vi "Parse GID_Telemetry.vi"(10 "Data In":variant) -> (2 "GID Telemetry":T1 {"Register_1"."A_Angle" format="%04x"; "Register_1"."B_Angle" format="%04x"; "Register_2"."Read_Time" format="%d ms"; "Register_2"."CMD_Code" format="%.0x"; "Register_2"."Head_Sel" format="%.0x"; "Register_7"."Spare" format="%04x"; "Register_8"."Spare" format="%04x"; "Register_A"."Spare" format="%04x"})   [LabVIEW 2019]
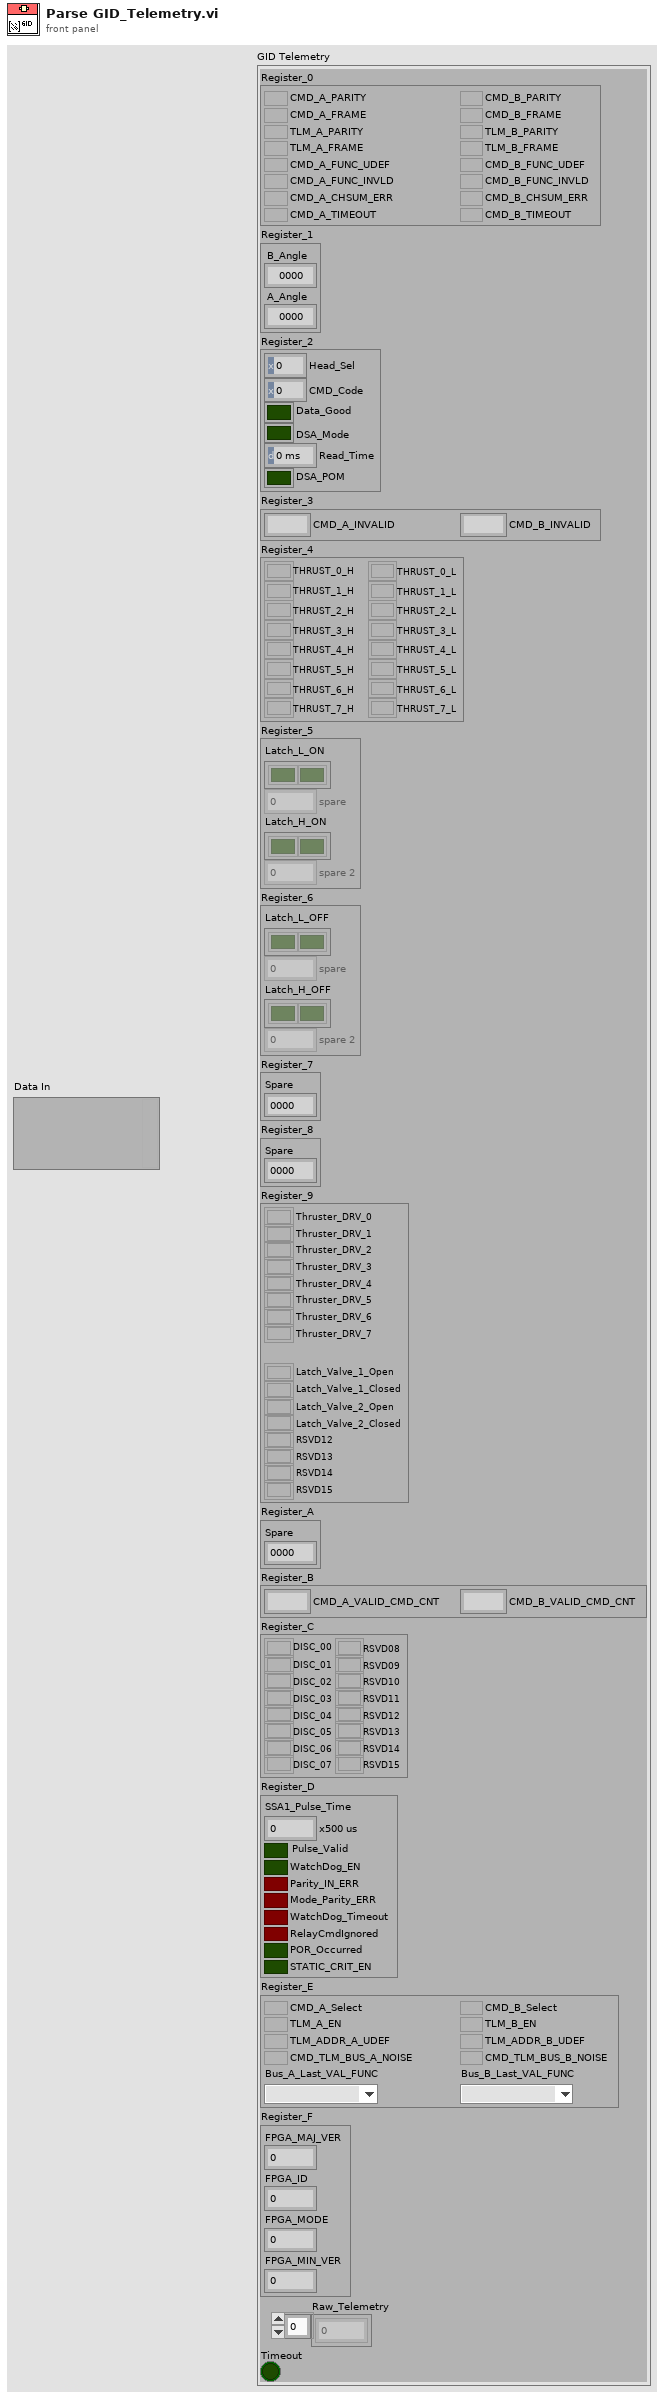
[diagram p1: front panel]
types:
  T1 = cluster{"Register_0":cluster{"CMD_B_PARITY":bool, "CMD_A_PARITY":bool, "CMD_B_FRAME":bool, "CMD_A_FRAME":bool, "TLM_B_PARITY":bool, "TLM_A_PARITY":bool, "TLM_B_FRAME":bool, "TLM_A_FRAME":bool, "CMD_B_FUNC_UDEF":bool, "CMD_A_FUNC_UDEF":bool, "CMD_B_FUNC_INVLD":bool, "CMD_A_FUNC_INVLD":bool, "CMD_B_CHSUM_ERR":bool, "CMD_A_CHSUM_ERR":bool, "CMD_B_TIMEOUT":bool, "CMD_A_TIMEOUT":bool}, "Register_1":cluster{"B_Angle":u8, "A_Angle":u8}, "Register_2":cluster{"Head_Sel":u8, "CMD_Code":u8, "Data_Good":bool, "DSA_Mode":bool, "Read_Time":u8, "DSA_POM":bool}, "Register_3":cluster{"CMD_B_INVALID":u8, "CMD_A_INVALID":u8}, "Register_4":cluster{"THRUST_0_H":bool, "THRUST_1_H":bool, "THRUST_2_H":bool, "THRUST_3_H":bool, "THRUST_4_H":bool, "THRUST_5_H":bool, "THRUST_6_H":bool, "THRUST_7_H":bool, "THRUST_0_L":bool, "THRUST_1_L":bool, "THRUST_2_L":bool, "THRUST_3_L":bool, "THRUST_4_L":bool, "THRUST_5_L":bool, "THRUST_6_L":bool, "THRUST_7_L":bool}, "Register_5":cluster{"Latch_L_ON":bool[], "spare":u8, "Latch_H_ON":bool[], "spare 2":u8}, "Register_6":cluster{"Latch_L_OFF":bool[], "spare":u8, "Latch_H_OFF":bool[], "spare 2":u8}, "Register_7":cluster{"Spare":u16}, "Register_8":cluster{"Spare":u16}, "Register_9":cluster{"Thruster_DRV_0":bool, "Thruster_DRV_1":bool, "Thruster_DRV_2":bool, "Thruster_DRV_3":bool, "Thruster_DRV_4":bool, "Thruster_DRV_5":bool, "Thruster_DRV_6":bool, "Thruster_DRV_7":bool, "Latch_Valve_1_Open":bool, "Latch_Valve_1_Closed":bool, "Latch_Valve_2_Open":bool, "Latch_Valve_2_Closed":bool, "RSVD12":bool, "RSVD13":bool, "RSVD14":bool, "RSVD15":bool}, "Register_A":cluster{"Spare":u16}, "Register_B":cluster{"CMD_B_VALID_CMD_CNT":u8, "CMD_A_VALID_CMD_CNT":u8}, "Register_C":cluster{"DISC_00":bool, "DISC_01":bool, "DISC_02":bool, "DISC_03":bool, "DISC_04":bool, "DISC_05":bool, "DISC_06":bool, "DISC_07":bool, "RSVD08":bool, "RSVD09":bool, "RSVD10":bool, "RSVD11":bool, "RSVD12":bool, "RSVD13":bool, "RSVD14":bool, "RSVD15":bool}, "Register_D":cluster{"SSA1_Pulse_Time":u8, "Pulse_Valid":bool, "WatchDog_EN":bool, "Parity_IN_ERR":bool, "Mode_Parity_ERR":bool, "WatchDog_Timeout":bool, "RelayCmdIgnored":bool, "POR_Occurred":bool, "STATIC_CRIT_EN":bool}, "Register_E":cluster{"CMD_B_Select":bool, "CMD_A_Select":bool, "TLM_B_EN":bool, "TLM_A_EN":bool, "TLM_ADDR_B_UDEF":bool, "TLM_ADDR_A_UDEF":bool, "CMD_TLM_BUS_B_NOISE":bool, "CMD_TLM_BUS_A_NOISE":bool, "Bus_B_Last_VAL_FUNC":enum16{"No_Command", "IO_Comand", "Latch_Valve", "Housekeeping", "Bad_Function"}, "Bus_A_Last_VAL_FUNC":enum16{"No_Command", "IO_Comand", "Latch_Valve", "Housekeeping", "Bad_Function"}}, "Register_F":cluster{"FPGA_MAJ_VER":u8, "FPGA_ID":u8, "FPGA_MODE":u8, "FPGA_MIN_VER":u8}, "Raw_Telemetry":u16[], "Timeout":bool}
  T2 = cluster{"Register_0":cluster{"CMD_B_PARITY":bool, "CMD_A_PARITY":bool, "CMD_B_FRAME":bool, "CMD_A_FRAME":bool, "TLM_B_PARITY":bool, "TLM_A_PARITY":bool, "TLM_B_FRAME":bool, "TLM_A_FRAME":bool, "CMD_B_FUNC_UDEF":bool, "CMD_A_FUNC_UDEF":bool, "CMD_B_FUNC_INVLD":bool, "CMD_A_FUNC_INVLD":bool, "CMD_B_CHSUM_ERR":bool, "CMD_A_CHSUM_ERR":bool, "CMD_B_TIMEOUT":bool, "CMD_A_TIMEOUT":bool}, "Register_1":cluster{"B_Angle":u8, "A_Angle":u8}, "Register_2":cluster{"Head_Sel":u8, "CMD_Code":u8, "Data_Good":bool, "DSA_Mode":bool, "Read_Time":u8, "DSA_POM":bool}, "Register_3":cluster{"CMD_B_INVALID":u8, "CMD_A_INVALID":u8}, "Register_4":cluster{"THRUST_0_H":bool, "THRUST_1_H":bool, "THRUST_2_H":bool, "THRUST_3_H":bool, "THRUST_4_H":bool, "THRUST_5_H":bool, "THRUST_6_H":bool, "THRUST_7_H":bool, "THRUST_0_L":bool, "THRUST_1_L":bool, "THRUST_2_L":bool, "THRUST_3_L":bool, "THRUST_4_L":bool, "THRUST_5_L":bool, "THRUST_6_L":bool, "THRUST_7_L":bool}, "Register_5":cluster{"Latch_L_ON":bool[], "spare":u8, "Latch_H_ON":bool[], "spare 2":u8}, "Register_6":cluster{"Latch_L_OFF":bool[], "spare":u8, "Latch_H_OFF":bool[], "spare 2":u8}, "Register_7":cluster{"Spare":u16}, "Register_8":cluster{"Spare":u16}, "Register_9":cluster{"Thruster_DRV_0":bool, "Thruster_DRV_1":bool, "Thruster_DRV_2":bool, "Thruster_DRV_3":bool, "Thruster_DRV_4":bool, "Thruster_DRV_5":bool, "Thruster_DRV_6":bool, "Thruster_DRV_7":bool, "Latch_Valve_1_Open":bool, "Latch_Valve_1_Closed":bool, "Latch_Valve_2_Open":bool, "Latch_Valve_2_Closed":bool, "RSVD12":bool, "RSVD13":bool, "RSVD14":bool, "RSVD15":bool}, "Register_A":cluster{"Spare":u16}, "Register_B":cluster{"CMD_B_VALID_CMD_CNT":u8, "CMD_A_VALID_CMD_CNT":u8}, "Register_C":cluster{"DISC_00":bool, "DISC_01":bool, "DISC_02":bool, "DISC_03":bool, "DISC_04":bool, "DISC_05":bool, "DISC_06":bool, "DISC_07":bool, "RSVD08":bool, "RSVD09":bool, "RSVD10":bool, "RSVD11":bool, "RSVD12":bool, "RSVD13":bool, "RSVD14":bool, "RSVD15":bool}, "Register_D":cluster{"SSA1_Pulse_Time":u8, "Pulse_Valid":bool, "WatchDog_EN":bool, "Parity_IN_ERR":bool, "Mode_Parity_ERR":bool, "WatchDog_Timeout":bool, "Spare":bool, "POR_Occurred":bool, "STATIC_CRIT_EN":bool}, "Register_E":cluster{"CMD_B_Select":bool, "CMD_A_Select":bool, "TLM_B_EN":bool, "TLM_A_EN":bool, "TLM_ADDR_B_UDEF":bool, "TLM_ADDR_A_UDEF":bool, "CMD_TLM_BUS_B_NOISE":bool, "CMD_TLM_BUS_A_NOISE":bool, "Bus_B_Last_VAL_FUNC":enum16{"No_Command", "IO_Comand", "Latch_Valve", "Housekeeping", "Bad_Function"}, "Bus_A_Last_VAL_FUNC":enum16{"No_Command", "IO_Comand", "Latch_Valve", "Housekeeping", "Bad_Function"}}, "Register_F":cluster{"FPGA_MAJ_VER":u8, "FPGA_ID":u8, "FPGA_MODE":u8, "FPGA_MIN_VER":u8}, "Raw_Telemetry":u16[], "Timeout":bool}
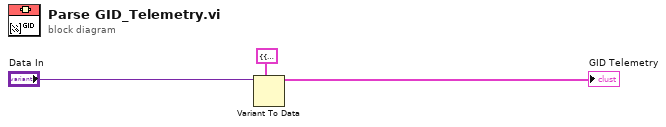
[diagram p0: block diagram]
diagram:
  n1 = Variant To Data(type=T2 {"Register_0"={"CMD_B_PARITY"=FALSE, "CMD_A_PARITY"=FALSE, "CMD_B_FRAME"=FALSE, "CMD_A_FRAME"=FALSE, "TLM_B_PARITY"=FALSE, "TLM_A_PARITY"=FALSE, "TLM_B_FRAME"=FALSE, "TLM_A_FRAME"=FALSE, "CMD_B_FUNC_UDEF"=FALSE, "CMD_A_FUNC_UDEF"=FALSE, "CMD_B_FUNC_INVLD"=FALSE, "CMD_A_FUNC_INVLD"=FALSE, "CMD_B_CHSUM_ERR"=FALSE, "CMD_A_CHSUM_ERR"=FALSE, "CMD_B_TIMEOUT"=FALSE, "CMD_A_TIMEOUT"=FALSE}, "Register_1"={"B_Angle"=0, "A_Angle"=0}, "Register_2"={"Head_Sel"=0, "CMD_Code"=0, "Data_Good"=FALSE, "DSA_Mode"=FALSE, "Read_Time"=0, "DSA_POM"=FALSE}, "Register_3"={"CMD_B_INVALID"=0, "CMD_A_INVALID"=0}, "Register_4"={"THRUST_0_H"=FALSE, "THRUST_1_H"=FALSE, "THRUST_2_H"=FALSE, "THRUST_3_H"=FALSE, "THRUST_4_H"=FALSE, "THRUST_5_H"=FALSE, "THRUST_6_H"=FALSE, "THRUST_7_H"=FALSE, "THRUST_0_L"=FALSE, "THRUST_1_L"=FALSE, "THRUST_2_L"=FALSE, "THRUST_3_L"=FALSE, "THRUST_4_L"=FALSE, "THRUST_5_L"=FALSE, "THRUST_6_L"=FALSE, "THRUST_7_L"=FALSE}, "Register_5"={"Latch_L_ON"=[], "spare"=0, "Latch_H_ON"=[], "spare 2"=0}, "Register_6"={"Latch_L_OFF"=[], "spare"=0, "Latch_H_OFF"=[], "spare 2"=0}, "Register_7"={"Spare"=0}, "Register_8"={"Spare"=0}, "Register_9"={"Thruster_DRV_0"=FALSE, "Thruster_DRV_1"=FALSE, "Thruster_DRV_2"=FALSE, "Thruster_DRV_3"=FALSE, "Thruster_DRV_4"=FALSE, "Thruster_DRV_5"=FALSE, "Thruster_DRV_6"=FALSE, "Thruster_DRV_7"=FALSE, "Latch_Valve_1_Open"=FALSE, "Latch_Valve_1_Closed"=FALSE, "Latch_Valve_2_Open"=FALSE, "Latch_Valve_2_Closed"=FALSE, "RSVD12"=FALSE, "RSVD13"=FALSE, "RSVD14"=FALSE, "RSVD15"=FALSE}, "Register_A"={"Spare"=0}, "Register_B"={"CMD_B_VALID_CMD_CNT"=0, "CMD_A_VALID_CMD_CNT"=0}, "Register_C"={"DISC_00"=FALSE, "DISC_01"=FALSE, "DISC_02"=FALSE, "DISC_03"=FALSE, "DISC_04"=FALSE, "DISC_05"=FALSE, "DISC_06"=FALSE, "DISC_07"=FALSE, "RSVD08"=FALSE, "RSVD09"=FALSE, "RSVD10"=FALSE, "RSVD11"=FALSE, "RSVD12"=FALSE, "RSVD13"=FALSE, "RSVD14"=FALSE, "RSVD15"=FALSE}, "Register_D"={"SSA1_Pulse_Time"=0, "Pulse_Valid"=FALSE, "WatchDog_EN"=FALSE, "Parity_IN_ERR"=FALSE, "Mode_Parity_ERR"=FALSE, "WatchDog_Timeout"=FALSE, "Spare"=FALSE, "POR_Occurred"=FALSE, "STATIC_CRIT_EN"=FALSE}, "Register_E"={"CMD_B_Select"=FALSE, "CMD_A_Select"=FALSE, "TLM_B_EN"=FALSE, "TLM_A_EN"=FALSE, "TLM_ADDR_B_UDEF"=FALSE, "TLM_ADDR_A_UDEF"=FALSE, "CMD_TLM_BUS_B_NOISE"=FALSE, "CMD_TLM_BUS_A_NOISE"=FALSE, "Bus_B_Last_VAL_FUNC"=enum."No_Command", "Bus_A_Last_VAL_FUNC"=enum."No_Command"}, "Register_F"={"FPGA_MAJ_VER"=0, "FPGA_ID"=0, "FPGA_MODE"=0, "FPGA_MIN_VER"=0}, "Raw_Telemetry"=[], "Timeout"=FALSE} ("GID Telemetry"), Variant="Data In") -> (data=→"GID Telemetry":T2)  [unwired: 1 in, 1 out]
